vi "flattenPlaneAngleToXML_Scalar.vi"(8 "error in (no error)":errorcluster, 9 "planeAngleUnitInXML":T1, 10 "planeAngleAgain":variant, 11 "planeAngle":dbl[unit]) -> (0 "error out":errorcluster, 3 "xmlString":string)   [LabVIEW 2016, in "UnitsAndXML.lvlib"]
uses:
  <userlib>/Common/UnitsAndXML/UnitsAndXML.lvlib
  <userlib>/Common/UnitsAndXML/FlattenItemWithUnitToXML/FlattenPlaneAngleToXML/PlaneAngleUnit.ctl
  <vilib>/Utility/VariantDataType/VariantType.lvlib
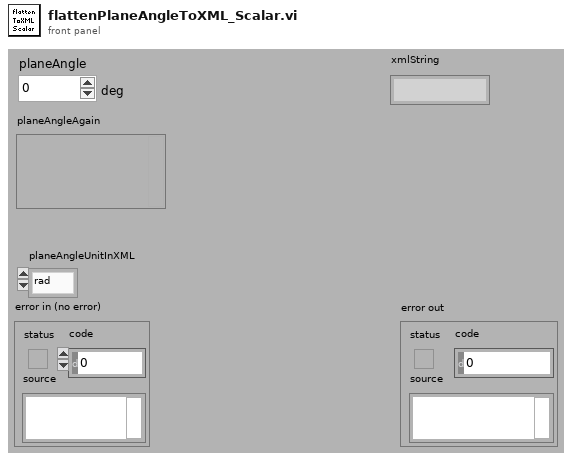
[diagram p1: front panel]
types:
  T1 = typedef "UnitsAndXML.lvlib/PlaneAngleUnit.ctl" = enum16{"rad", "deg", "'", "\""}
  T2 = typedef "VariantType.lvlib/Type.ctl" = enum8{"Invalid Type", "Void", "I8", "I16", "I32", "I64", "U8", "U16", "U32", "U64", "Single Float", "Double Float", "Extended Float", "Single Complex", "Double Complex", "Extended Complex", "Enum U8", "Enum U16", "Enum U32", "Enum U64", "Single Float With Unit", "Double Float With Unit", "Extended Float With Unit", "Single Complex with Unit", "Double Complex with Unit", "Extended Complex with Unit", "Boolean", "String", "Path", "Picture", "Tag", "Array", "Cluster", "Variant", "LV Variant", "Waveform", "Timestamp", "Digital Waveform", "Digital Data", "ExpressData", "Refnum", "External Data", "VI", "Poly VI", "LabVIEW Class Instance", "Fixed Point"}
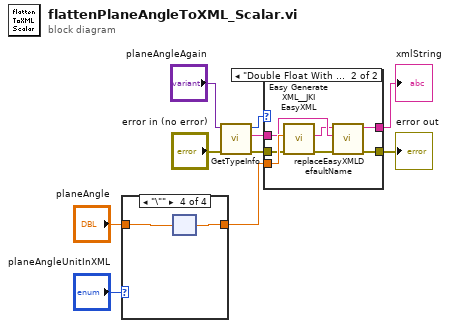
[diagram p0: block diagram]
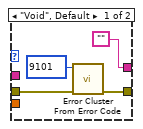
[diagram p2: hidden frame]
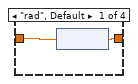
[diagram p3: hidden frame]
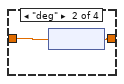
[diagram p4: hidden frame]
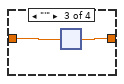
[diagram p5: hidden frame]
diagram:
  n1 = case shown="\"\\\"\"" "planeAngleUnitInXML" {
    tunnel: "planeAngle" -> [w12 w14 w16 w18]
    tunnel: [w11 w13 w15 w17] -> w10
    frame "rad", Default {
      n2 = node(w12) -> (w11:dbl)
    }
    frame "deg" {
      n3 = node(w14) -> (w13:dbl)
    }
    frame "'" {
      n4 = node(w16) -> (w15:dbl)
    }
    frame "\"" {
      n5 = node(w18) -> (w17:dbl)
    }
  }
  n6 = call <vilib>:"GetTypeInfo.vi"("error in (no error)"="error in (no error)", "Variant"="planeAngleAgain") -> ("error out"=w2:errorcluster, "Name"=w1:string, "Type Enum"=w3:T2)  [unwired: 5 in, 2 out]
  n7 = case shown="\"Double Float With Unit\"" w3 {
    tunnel: w10 -> [_ w29]
    tunnel: ["" w28] -> w7
    tunnel: [w21 w27] -> w6
    tunnel: w2 -> [w19 w24]
    tunnel: w1 -> [_ w26]
    frame "Void", Default {
      n8 = call <vilib>:"Error Cluster From Error Code.vi"("error in (no error)"=w19, "error code (0)"=9101) -> ("error out"=w21:errorcluster)  [unwired: 7 in]
    }
    frame "Double Float With Unit" {
      n9 = call <vilib>:"Easy Generate XML__JKI EasyXML.vi"("error in (no error)"=w24, "LabVIEW Data"=w29) -> ("error out"=w23:errorcluster, "XML String"=w25:string)  [unwired: 8 in]
      n10 = call <userlib>:"replaceEasyXMLDefaultName.vi"("error in"=w23, "desiredName"=w26, "easyXMLStringWithDefaultNames"=w25) -> ("error out"=w27:errorcluster, "xmlString"=w28:string)  [unwired: 7 in]
    }
  }
  "xmlString" <- w7
  "error out" <- w6
